vi "Initialize FPGA values.vi"(8 "Error In":errorcluster) -> (0 "Error Out":errorcluster, 3 "AOL_Globals":T1={"Imaging Protocol"=enum."Live Imaging", "Number of POI"=0, "Number of Miniscans"=0, "Number of Trials"=0, "Number of Cycles "=0, "# Averaged Frames"=0, "Laser power (%)"=0, "Pockels (V)"=0.0, "Acquisition Length (sec)"=0.0, "Fill time (us)"=0.0, "POI Dwell time (us)"=0.0, "Miniscan Dwell time per pixel (us)"=0.0, "PMT 1"=0.0, "PMT 2"=0.0, "Back Apperture (mA)"=0.0, "Frame Size"=200, "Center Frequency"=0.0, "Field of View (um)"=175.0, "Field of View (norm)"=0.0, "DwellTime (us)"=0.0, "Ref Dwell Time (us)"=0.0, "Wavelength (nm)"=0.0, "Zoom"=0.0, "AOL Z"=0.0, "AOL Mode"=enum."Raster", "GridXY"=0.0, "GridZ"=0.0, "TriggerPeriod (sec)"=0.0, "Number of Pixels in Miniscan"=0, "Experiment folder path"=path "", "X centre"=0.0, "Y centre"=0.0, "Angle (degrees)"=0.0, "Angle Xs (degrees)"=0.0, "Angle Ys (degrees)"=0.0, "Plane Mode"=0, "Threshold"=[], "Regenerate Chirps"=FALSE, "Rectangle ROI length (pixels)"=0, "Rectangle ROI height (pixels)"=0, "AOD fill"=4900, "StartupDelay"=0, "Samples Wait after Trigger"=5080, "Slip Cycle"=600000, "Add Cycle"=TRUE, "Functional Mode"=enum."Point", "Z Start"=0.0, "Z Stop"=0.0, "# Planes"=0, "Total Pixels"=0, "Variable Miniscan Pixels"=[], "Use Variable Length"=FALSE, "Use Variable Resolution"=FALSE, "Laser power (%) at Z Start"=0, "Laser power (%) at Z Stop"=0, "Ref Z Step"=0} {"Angle Ys (degrees)" format="%#.6g"; "Angle Xs (degrees)" format="%#.6g"; "Plane Mode" items=["XY Plane", "XZ Plane", "YZ Plane", "arbitraryplane"]; "Frame Size" items=["100X100"=100, "128X128"=128, "200X200"=200, "256X256"=256, "512X512"=512, "1024x1024"=1024, "2048x2048"=2048]; "Back Apperture (mA)" format="%#.6g"; "Pockels (V)" format="%#.6g"; "PMT 2" format="%#.6g"; "PMT 1" format="%#.6g"; "Angle (degrees)" format="%#.6g"; "POI Dwell time (us)" format="%#.6g"})   [LabVIEW 2020]
uses:
  Typedefs/Controls/AOL_Globals.ctl
  Typedefs/Imaging Protocols enum.ctl
  Typedefs/Frame Size.ctl
  Typedefs/AOL modes.ctl
  Typedefs/Plane Mode.ctl
  Typedefs/Functional Mode.ctl
  Typedefs/HW config states enum.ctl
panel:
  # "To be integrated to one of the FGVs and read/write to file."
  # "Non-MovCor parameters"
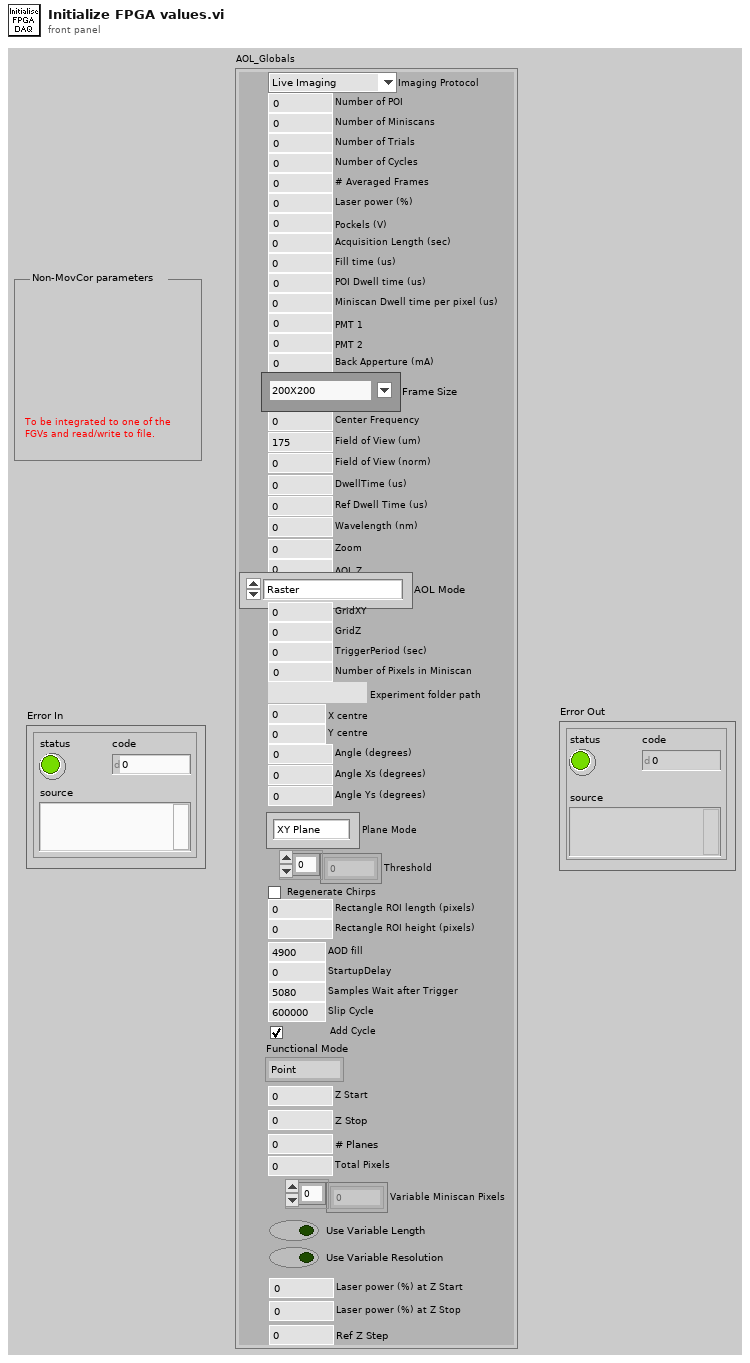
[diagram p1: front panel]
types:
  T1 = typedef "AOL_Globals.ctl" = cluster{"Imaging Protocol":T2, "Number of POI":u16, "Number of Miniscans":u16, "Number of Trials":u16, "Number of Cycles ":u64, "# Averaged Frames":u16, "Laser power (%)":u8, "Pockels (V)":dbl, "Acquisition Length (sec)":dbl, "Fill time (us)":dbl, "POI Dwell time (us)":dbl, "Miniscan Dwell time per pixel (us)":dbl, "PMT 1":dbl, "PMT 2":dbl, "Back Apperture (mA)":dbl, "Frame Size":T3, "Center Frequency":dbl, "Field of View (um)":dbl, "Field of View (norm)":dbl, "DwellTime (us)":dbl, "Ref Dwell Time (us)":dbl, "Wavelength (nm)":dbl, "Zoom":dbl, "AOL Z":dbl, "AOL Mode":T4, "GridXY":dbl, "GridZ":dbl, "TriggerPeriod (sec)":dbl, "Number of Pixels in Miniscan":u16, "Experiment folder path":path, "X centre":dbl, "Y centre":dbl, "Angle (degrees)":dbl, "Angle Xs (degrees)":dbl, "Angle Ys (degrees)":dbl, "Plane Mode":T5, "Threshold":u16[], "Regenerate Chirps":bool, "Rectangle ROI length (pixels)":u16, "Rectangle ROI height (pixels)":u16, "AOD fill":u16, "StartupDelay":i32, "Samples Wait after Trigger":u16, "Slip Cycle":u32, "Add Cycle":bool, "Functional Mode":T6, "Z Start":dbl, "Z Stop":dbl, "# Planes":i32, "Total Pixels":i32, "Variable Miniscan Pixels":u16[], "Use Variable Length":bool, "Use Variable Resolution":bool, "Laser power (%) at Z Start":u8, "Laser power (%) at Z Stop":u8, "Ref Z Step":i8}
  T2 = typedef "Imaging Protocols enum.ctl" = enum16{"AOL Z-Stack", "Motor Z Stack", "Parameter Sweep", "Functional Acquisition", "Single Plane Acquisition", "Volume Acquisition", "Live Imaging", "Live Plane Imaging", "Live Volume Imaging"}
  T3 = typedef "Frame Size.ctl" = u16
  T4 = typedef "AOL modes.ctl" = enum16{"Raster", "Structural", "Pointing", "Mini Scan", "Alignment"}
  T5 = typedef "Plane Mode.ctl" = u16
  T6 = typedef "Functional Mode.ctl" = enum16{"Point", "Line", "Patch", "Plane", "Volume"}
  T7 = typedef "HW config states enum.ctl" = enum16{"Load from file", "Save to file", "Save backup", "Write all", "Read all", "Write XY stage settings", "Write DAQ FPGA settings", "Write Control FPGA settings", "Write Phys Channels", "Write System Config", "Write HW Config", "Save System Config", "Save HW Config", "Clear", "Compare from file"}
  T8 = typedef "Hardware Configuration settings.ctl" = cluster{"Dev. PC":bool, "Swap XY on stage":bool, "No of AOD":u8, "MC Supported":bool, "Axial MC":bool, "Computer MAC address":string, "Externalise Triggers":bool, "Trigger HW config":T9, "DAQmx Chan":T10, "XYZ Stage Control Config":T11, "XY stage available":bool, "XY Comms Config Cluster":T12, "Y stage available":bool, "Y Comms Config Cluster":T12, "Z stage available":bool, "Z Comms Config Cluster ":T12, "Encoder available":bool, "Encoder":T14, "VidRec available":bool, "Cam VidRec":T15, "Laser Power Control HW config":T16, "Laser 1 available":bool, "Laser 1 config cluster":T17, "Prechirper 1 available":bool, "Prechirper 1 config cluster":T18, "Control system.FPGA available?":bool, "Control Sys. HW config":T19, "DAQ FPGA HW Config":T20, "PMT Control Voltage Limits":T24}
  T9 = typedef "Triggers HW config.ctl" = cluster{"Available Device List":i32, "Device Address":string}
  T10 = typedef "DAQmx physical channels cluster.ctl" = cluster{"Pockels AO":tag, "Hard shutter AO":tag, "PMT AOs":tag, "Galvo AOs":tag, "Power meter AI":tag}
  T11 = typedef "XYZControlConfig.ctl" = enum16{"None", "XYZ", "XY-Z", "X-Y-Z", "Z"}
  T12 = typedef "Peripherals comms config cluster.ctl" = cluster{"Name":string, "Device Address":string, "Port ":u16, "Baudrate":i32, "Comms Type":T13}
  T13 = typedef "Comms Type.ctl" = enum16{"GPIB-IEEE488", "Serial-RS232", "Serial-RS485", "Serial-RS422", "Serial-USB", "Ethernet-TCP/IP", "Ethernet-UDP"}
  T14 = typedef "Encoder config cluster.ctl" = cluster{"IP address":string, "Port":u16, "Wheel radius (cm)":dbl, "Encoder Trigger":tag}
  T15 = typedef "Cam VidRec HW config setup cluster.ctl" = cluster{"DO flag-Video record":tag, "DO flag-Trial start":tag}
  T16 = typedef "Laser Power Control HW config.ctl" = cluster{"Laser Power Control":string, "Laser Power Modulation Control":enum16{"NI", "FPGA"}}
  T17 = typedef "Laser 1 config cluster.ctl" = cluster{"COM port":refnum<visa-resource-name>, "Baud Rate":i32, "Type":string}
  T18 = typedef "PreChirper 1 config cluster.ctl" = cluster{"Type":string, "Baud Rate":i32, "COM port":refnum<visa-resource-name>}
  T19 = typedef "Control Sys HW config cluster.ctl" = cluster{"Control system.FPGA Type":enum16{"Virtex 5", "Virtex 7"}, "Control system.Network adapter name":string, "Control system.MAC address":string, "Control system.Ethernet Port":u32, "Control system.Ethernet Port Opened":bool}
  T20 = typedef "DAQ FPGA HW config cluster.ctl" = cluster{"FGPA Ref":T21, "Target":T22, "input card type":T23}
  T21 = typedef "FPGA Ref.ctl" = refnum<k20>
  T22 = typedef "nirio_resource_hc.ctl" = tag
  T23 = typedef "FPGA input type AC-DC.ctl" = enum16{"AC Card", "DC Card"}
  T24 = typedef "PMT Control Voltage limits.ctl" = cluster{"Lower Limit":dbl, "Upper Limit":dbl}
  T25 = typedef "DAQ Input Parameters(FlexRIO).ctl" = cluster{"Mode":T26, "Zoom":i8, "Acceptance Angle":i8, "AOD fill":u16, "Wavelength":i16, "Speed of Sound(Va)":i8, "Samps-per-pix(P)":i16, "Numer-pixels-pointing(Np)":u32, "Samples Wait after Trigger":u16, "StartUp Delay":i32, "x-pixels-per-line(NPx) (fast)":u16, "y-pixels-per-line(NPy) (slow)":u16, "Repeat (Number of Cycles)":u32, "Number of Trials":u16, "Ref threshold":u16, "Slip Cycle":u32, "proportioanl_scale":fxp<+,16,2>, "Ref Average":u16, "Sliding Average":bool, "Integral_scale":fxp<+/-,16,12>, "diff_thresh":fxp<+/-,16,8>, "diff_threshZ":fxp<+/-,16,8>, "lines_for_2ms":i16, "Use accumulate green":bool, "Use accumulate red":bool, "Add Cycle":bool, "Ref Samps-per-pix(Pr)":i16, "Ref X-pixels-per-line(Npxr)":i16, "Ref Y-pixels-per-line(NPyr)":i16, "Ref_Z_Lines":i16, "Ref Scan Cycles":i32, "scale":fxp<+,16,2>, "accn_noise":fxp<+,16,16>, "var_y":fxp<+,16,4>, "var_x":fxp<+,16,4>, "New line trigger enabled":bool, "Ref count reset enabled":bool, "Control algorithm":T27, "proportioanl_scale Z":fxp<+,16,2>, "Integral_scale Z":fxp<+/-,16,12>, "Variable Miniscan Pixels":u16[], "Use Variable Length":bool}
  T26 = typedef "scan_type.ctl" = enum16{"Scanning", "Pointing", "Pointing & MC", "Scanning & MC"}
  T27 = typedef "Control algorithm.ctl" = enum16{"PID", "Kalman"}
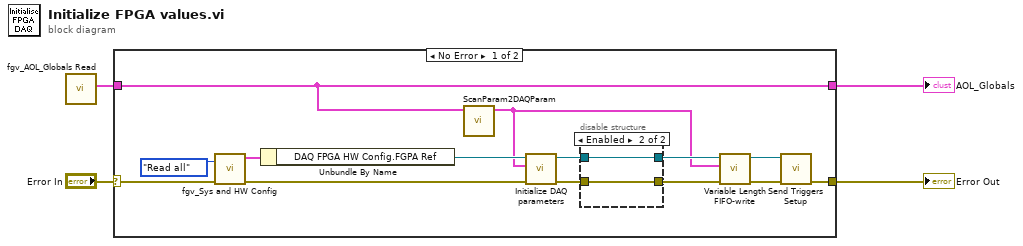
[diagram p0: block diagram]
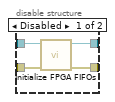
[diagram p2: hidden frame]
diagram:
  n1 = call "fgv_AOL_Globals Read.vi"() -> ("AOL_Globals"=w1:T1)  [unwired: 9 in, 2 out]
  n2 = case shown="No Error" "Error In" {
    selector: "Error In" -> [w14 w25]
    tunnel: [w17 w25] -> w3
    tunnel: [w18 w26] -> w2
    tunnel: w1 -> [w18 w26]
    frame No Error {
      n3 = call "fgv_Sys and HW Config.vi"("Function"=HW_config_states_enum."Read all", "error in (no error)"=w14) -> ("error out"=w13:errorcluster, "Hardware Configuration OUT"=w12:T8)  [unwired: 7 in, 1 out]
      n4 = Unbundle By Name(w12) -> ("DAQ FPGA HW Config.FGPA Ref"=w15:T21)
      n5 = call "ScanParam2DAQParam.vi"("AOL_Globals"=w18) -> ("DAQ Input Parameters(FlexRIO)"=w5:T25)  [unwired: 9 in, 1 out]
      n6 = call "Initialize DAQ parameters.vi"("error in"=w13, "DAQ Input Parameters(FlexRIO)"=w5, "FPGA VI Reference"=w15) -> ("error out"=w10:errorcluster, "FPGA VI Reference"=w11:T21)  [unwired: 7 in]
      n7 = disable-structure shown="Enabled" {
        disable-tunnel: w11 -> [w22 w24]
        disable-tunnel: w10 -> [w21 w23]
        disable-tunnel: [w20 w23] -> w9
        disable-tunnel: [w19 w24] -> w7
        frame Disabled {
          n8 = call "Initialize FPGA FIFOs.vi"("error in (no error)"=w21, "FGPA Ref"=w22) -> ("error out"=w20:errorcluster, "FGPA Ref"=w19:T21)  [unwired: 8 in]
        }
        frame Enabled {
        }
      }
      n9 = call "Variable Length FIFO-write.vi"("error in (no error)"=w9, "DAQ Input Parameters(FlexRIO)"=w5, "FGPA Ref"=w7) -> ("error out"=w8:errorcluster, "FGPA Ref"=w6:T21)  [unwired: 7 in]
      n10 = call "Send Triggers Setup.vi"("error in (no error)"=w8, "FGPA Ref"=w6) -> ("error out"=w17:errorcluster)  [unwired: 8 in, 1 out]
    }
    frame Error {
    }
  }
  "Error Out" <- w3
  "AOL_Globals" <- w2
